vi "Init Magnet Calibration.vi"(0 "Magnet Id":string) -> (1 "Calibration":T1={"Current Scale Factor kA/V"=1.0, "I->B"=[0.0, 1.0, 0.0], "B->I"=[0.0, 1.0, 0.0]} {"B->I" format="%.5e"; "Current Scale Factor kA/V" format="%.2f"; "I->B" format="%.5e"}, 2 "Error Code":i32, 3 "Error message":string)   [LabVIEW 2021]
doc: "This VI reads a magnet calibration file for the coefficients to convert kA to tesla.\nScott Hannahs, FBNML, Jan 1992"
uses:
  Serial Instruments/Power Supplies/PS Comm Globals.vi
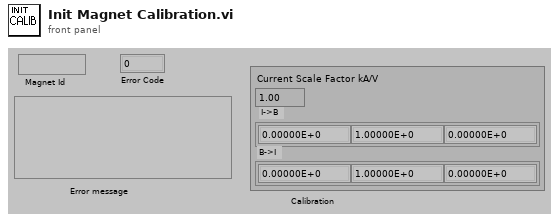
[diagram p1: front panel]
types:
  T1 = cluster{"Current Scale Factor kA/V":dbl, "I->B":dbl[], "B->I":dbl[]}
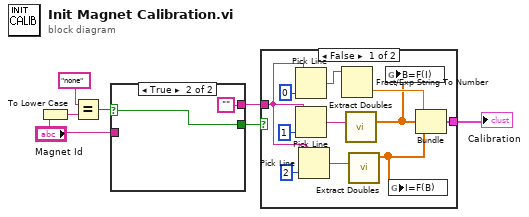
[diagram p0: block diagram]
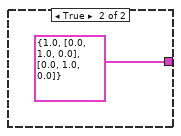
[diagram p2: hidden frame]
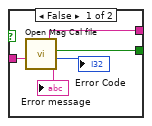
[diagram p3: hidden frame]
diagram:
  n1 = To Lower Case(string="Magnet Id") -> (all lower case string=w5:string)
  n2 = Equal?(x="none", y=w5) -> (x = y?=w2:bool)
  n3 = case shown="True" w2 {
    selector: w2 -> [_ w14]
    tunnel: "Magnet Id" -> [w12 _]
    tunnel: [w9 w14] -> w1
    tunnel: [w8 ""] -> w3
    frame False {
      n4 = call "Open Mag Cal file.vi"("Magnet Id"=w12) -> ("String"=w8:string, "Error"=w9:bool, "Error Code"=→"Error Code":i32, "Error message"=→"Error message":string)
    }
    frame True {
    }
  }
  n5 = case shown="False" w1 {
    tunnel: [w23 cluster{dbl, dbl[], dbl[]} {1.0, [0.0, 1.0, 0.0], [0.0, 1.0, 0.0]}] -> w4
    tunnel: w3 -> [w15 _]
    frame False {
      n6 = Pick Line(multi-line string=w15, line index=0) -> (output string=w24:string)  [unwired: 1 in]
      n7 = Pick Line(multi-line string=w15, line index=1) -> (output string=w25:string)  [unwired: 1 in]
      n8 = Pick Line(multi-line string=w15, line index=2) -> (output string=w18:string)  [unwired: 1 in]
      n9 = Fract/Exp String To Number(string=w24) -> (number=w22:dbl)  [unwired: 3 in, 1 out]
      n10 = call "Extract Doubles.vi"("String"=w25) -> ("Data"=w17:dbl[])  [unwired: 5 in, 1 out]
      n11 = call "Extract Doubles.vi"("String"=w18) -> ("Data"=w16:dbl[])  [unwired: 5 in, 1 out]
      n12 = global write "PS Comm Globals.vi" "B=F(I)"(w17) -> ()
      n13 = global write "PS Comm Globals.vi" "I=F(B)"(w16) -> ()
      n14 = Bundle(w22, "Data"=w17, "Data"=w16) -> (w23:cluster{dbl, "Data":dbl[], "Data":dbl[]})  [unwired: 1 in]
    }
    frame True {
    }
  }
  "Calibration" <- w4
